vi "Cell color by inspection (1D).vi"(4 "행번호":i32, 5 "Spec":dbl[](array[numeric]), 7 "Data (DBL)":dbl[](array[numeric]), 8 "에러 입력":errorcluster caption="에러 입력(에러 없음)", 9 "테이블 입력":refnum<vi>, 11 "Data (str)":string[](array[string])) -> (0 "에러 출력":errorcluster)   [LabVIEW 2020]
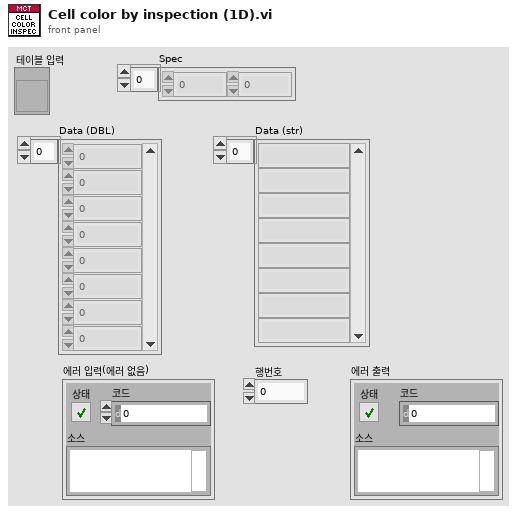
[diagram p1: front panel]
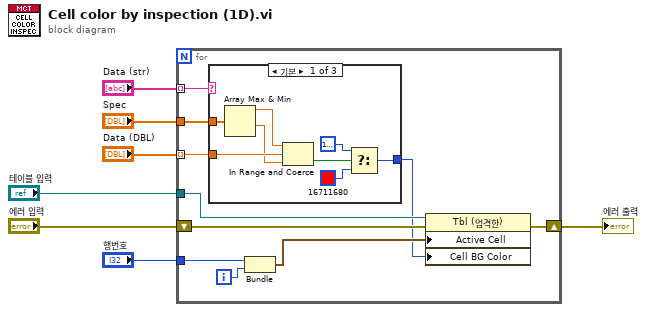
[diagram p0: block diagram]
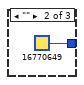
[diagram p2: hidden frame]
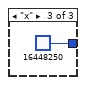
[diagram p3: hidden frame]
diagram:
  n1 = for {
    tunnel: "Spec" -> [w8]
    tunnel: "Data (DBL)" -> [w9] mode=indexing
    tunnel: "테이블 입력" -> [w17]
    tunnel: "Data (str)" -> [w10] mode=indexing
    tunnel: "행번호" -> [w16]
    shift-right: [w12] -> w7
    shift-left: "에러 입력" -> [w13]
    i -> [w15]
    n2 = case shown="기본" w10 {
      tunnel: w9 -> [w25 _ _]
      tunnel: [w22 u32 16770649 u32 16448250] -> w11
      tunnel: w8 -> [w20 _ _]
      frame Default {
        n3 = Array Max & Min(array=w20) -> (max value=w19:dbl, min value=w18:dbl)  [unwired: 2 out]
        n4 = In Range and Coerce(upper limit=w19, x=w25, lower limit=w18) -> (In Range?=w24:bool)  [unwired: 1 out]
        n5 = Select(t=u32 16777226, s=w24, f=u32 16711680) -> (s? t:f=w22:u32)
      }
      frame "" {
      }
      frame "ⅹ" {
      }
    }
    n6 = Bundle("행번호"=w16, w15) -> (w14:cluster{"행번호":i32, i32})  [unwired: 1 in]
    n7 = property class="Tbl (엄격한)"(reference=w17, error in=w13, "Active Cell"=w14, "Cell BG Color"=w11) -> (error out=w12:errorcluster)  [unwired: 1 out]
  }
  "에러 출력" <- w7
